vi "InitiateBurstModeRoutedMessage_Parse.vi"(8 "error in (no error)":errorcluster, 11 "message":variant) -> (0 "error out":errorcluster, 2 "InitiateBurstMode":T1)   [LabVIEW 2017, in "BurstMode.lvlib"]
uses:
  <vilib>/addons/InsightCM/Devices/Shared/Cms/CmsBurstMode/BurstMode.lvlib
  <vilib>/addons/InsightCM/Devices/Shared/Cms/CmsBurstMode/controls/InitiateBurstMode.ctl
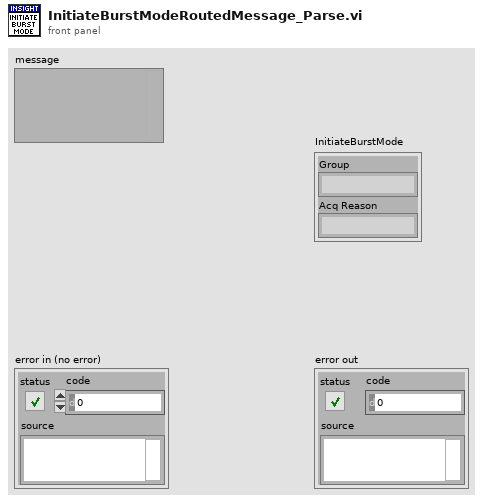
[diagram p1: front panel]
types:
  T1 = typedef "BurstMode.lvlib/InitiateBurstMode.ctl" = cluster{"Group":string, "Acq Reason":string}
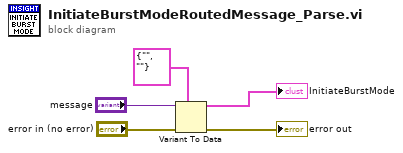
[diagram p0: block diagram]
diagram:
  n1 = Variant To Data(error in="error in (no error)", type=T1 {"Group"="", "Acq Reason"=""} ("InitiateBurstMode"), Variant="message") -> (data=→"InitiateBurstMode":T1, error out=→"error out":errorcluster)
